vi "Read Singleton.vi"(8 "error in (no error)":errorcluster) -> (0 "error out":errorcluster, 2 "Object Data Out":refnum<class>)   [LabVIEW 2020, in "Singleton.lvlib"]
uses:
  Singleton.lvlib
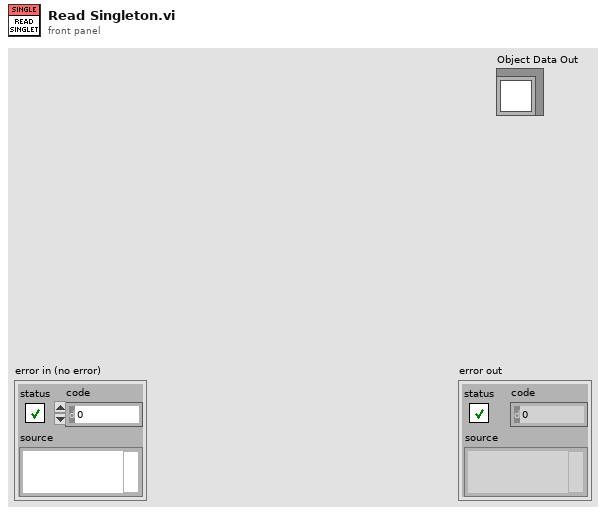
[diagram p1: front panel]
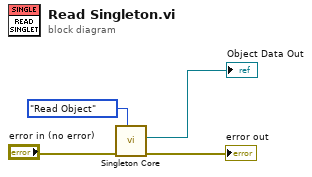
[diagram p0: block diagram]
diagram:
  n1 = call "Singleton Core.vi"("Action"=enum16{"Init", "Write Object", "Read Object"}."Read Object", "error in (no error)"="error in (no error)") -> ("error out"=→"error out":errorcluster, "Class out"=→"Object Data Out":refnum<class>)  [unwired: 8 in]
